vi "Sign Convention.vi"(9 "intake speed":dbl, 10 "grid-dy commands":T2, 11 "current object":T1=enum."cube") -> (2 "new object":T1, 3 "sign convention value":dbl)   [LabVIEW 2020]
uses:
  manipulator/Implementation/Typedefs/the grid-dy.ctl
  manipulator/Implementation/Typedefs/game object.ctl
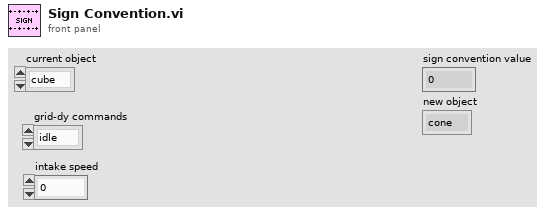
[diagram p1: front panel]
types:
  T1 = typedef "game object.ctl" = enum16{"cone", "cube"}
  T2 = typedef "the grid-dy.ctl" = enum16{"idle", "intake cone", "intake cube", "score low cone outtake", "score low cube outtake", "score mid cone", "score mid cube", "score high cone", "score high cube"}
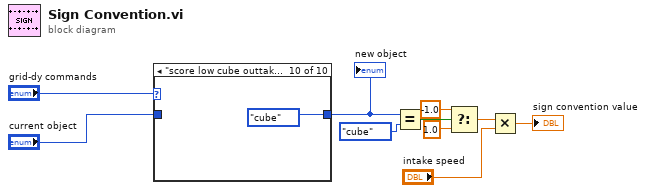
[diagram p0: block diagram]
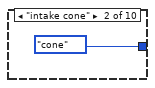
[diagram p3: hidden frame]
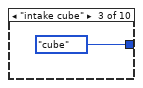
[diagram p4: hidden frame]
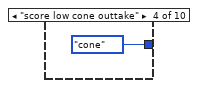
[diagram p5: hidden frame]
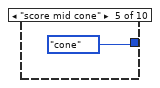
[diagram p6: hidden frame]
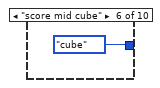
[diagram p7: hidden frame]
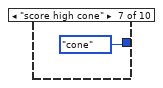
[diagram p8: hidden frame]
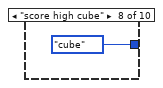
[diagram p9: hidden frame]
diagram:
  n1 = case shown="\"score low cube outtake\"" "grid-dy commands" {
    tunnel: [w11 game_object."cone" game_object."cube" ("y") game_object."cone" ("y") game_object."cone" ("y") game_object."cube" ("y") game_object."cone" ("y") game_object."cube" ("y") w19 game_object."cube" ("y")] -> w8
    tunnel: "current object" -> [w11 _ _ _ _ _ _ _ w19 _]
    frame Default {
    }
    frame "intake cone" {
    }
    frame "intake cube" {
    }
    frame "score low cone outtake" {
    }
    frame "score mid cone" {
    }
    frame "score mid cube" {
    }
    frame "score high cone" {
    }
    frame "score high cube" {
    }
    frame "idle" {
    }
    frame "score low cube outtake" {
    }
  }
  "new object" <- w8
  n2 = Equal?(x=w8, y=game_object."cube") -> (x = y?=w10:bool)
  n3 = Select(t=-1.0, s=w10, f=1.0) -> (s? t:f=w6:dbl)
  n4 = Multiply(x=w6, y="intake speed") -> (x*y=→"sign convention value":dbl)
